vi "gl_Time series viewer globals.vi"() -> ()   [LabVIEW 2013]
uses:
  Typedefs/Timelapse viewer refs.ctl
  Typedefs/Custom slider-horisontal.ctl
  Typedefs/AVI playback header info cluster.ctl
  Typedefs/AVI modes refs cluster.ctl
  <vilib>/vision/Avi1.llb/AviRefnum.ctl
  <vilib>/vision/Avi.llb/IMAQ AVI2 Refnum.ctl
panel:
  out "Funct viewer bring to front":bool
  out "Funct viewer window is open":bool
  out "Intensity":T1={0.0, 4095.0} scale=0.0..4095.0
  in  "Cursor.PosY":dbl=304.0
  in  "Start/End frame":T2
  in  "Speed graph length (s)":i32=10
  out "Window is open":bool
  out "Bring to front":bool
  in  "Use manual FPS?":bool
  in  "Manual frame rate (FPS)":dbl=30.0
  in  "Layout change":bool
  in  "Window 4 bring to front":bool
  in  "Window 3 bring to front":bool
  in  "Window 2 bring to front":bool
  in  "Window 1 bring to front":bool
  in  "Close larger image windows":bool
  in  "Video in larger window":string
  in  "Speed chart history length":i32=304
  out "AVI modes refs":T3
  out "1021th frame":bool
  in  "AVI base filenames":string[](array[string])=["Red Channel", "Green Channel"]
  out "# of Frames":u32
  in  "Playback speed mult.":dbl=1.0 step=0.1
  in  "Speed acquisition rate (ms)":dbl=2.0 format="%#_13g"
  in  "AVI playback header info cluster":T6={"Frame Size"=512, "AOD fill time (us)"=1.0, "Dwell time (us)"=24.5, "Frame period (ms)"=33.0, "Number of Miniscans"=0, "Number of Pixels in Miniscan"=0}
  in  "Timelapse viewer refs":T7
  # "This is the chart history length.\nThe Patch acq viewer was upgraded to set this global variable automatically.\nThe timelapse viewer still needs upgrading in the same way as the Patch acq viewer."
  # "Used by the temporary \n\"Window-Functional data editor.vi\""
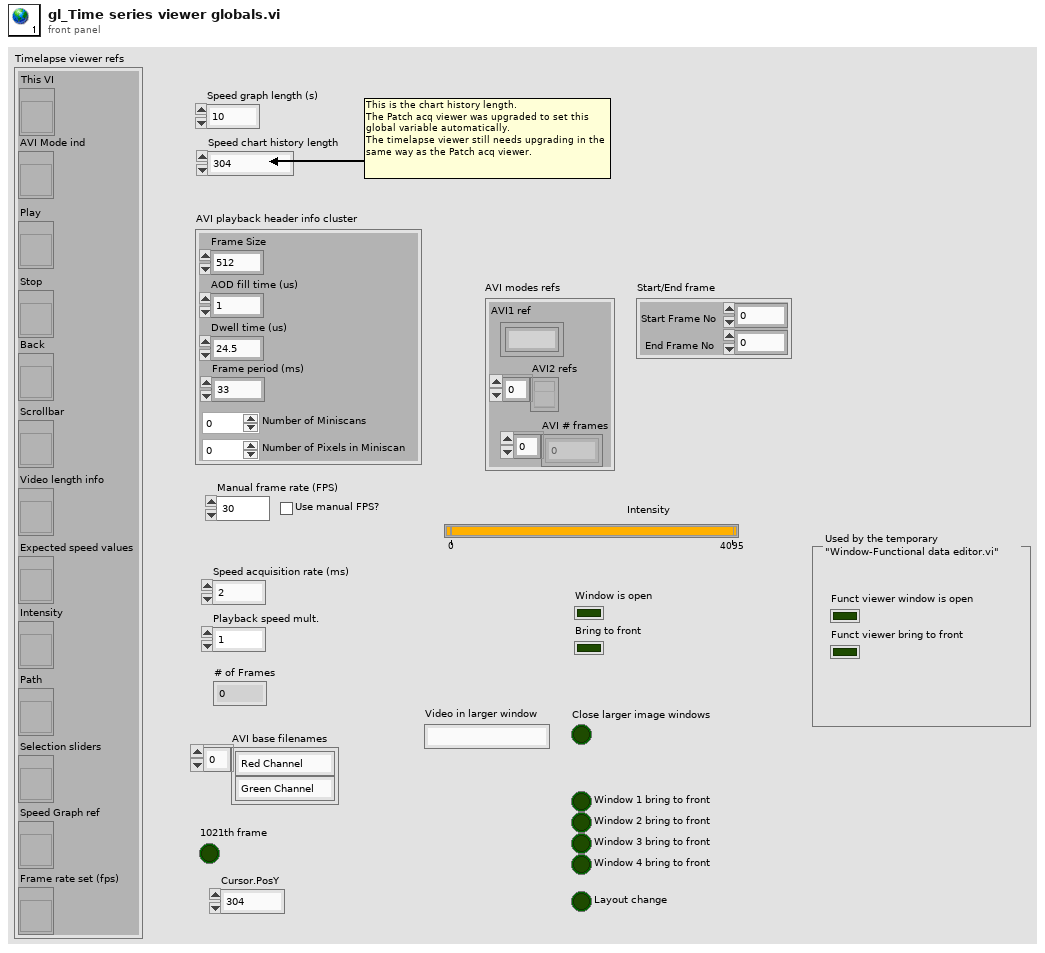
[diagram p1: front panel]
types:
  T1 = typedef "Custom slider-horisontal.ctl" = cluster{dbl, dbl}
  T2 = cluster{"Start Frame No":i32, "End Frame No":i32}
  T3 = typedef "AVI modes refs cluster.ctl" = cluster{"AVI1 ref":T4, "AVI2 refs":T5[], "AVI # frames":u32[]}
  T4 = typedef "AviRefnum.ctl" = refnum<k1>
  T5 = typedef "IMAQ AVI2 Refnum.ctl" = refnum<k20>
  T6 = typedef "AVI playback header info cluster.ctl" = cluster{"Frame Size":u32, "AOD fill time (us)":dbl, "Dwell time (us)":dbl, "Frame period (ms)":dbl, "Number of Miniscans":u16, "Number of Pixels in Miniscan":u16}
  T7 = typedef "Timelapse viewer refs.ctl" = cluster{"This VI":refnum<vi>, "AVI Mode ind":refnum<vi>, "Play":refnum<vi>, "Stop":refnum<vi>, "Back":refnum<vi>, "Scrollbar":refnum<vi>, "Video length info":refnum<vi>, "Expected speed values":refnum<vi>, "Intensity":refnum<vi>, "Path":refnum<vi>, "Selection sliders":refnum<vi>, "Speed Graph ref":refnum<vi>, "Frame rate set (fps)":refnum<vi>}
diagram:
